vi "02_Stat_Read.vi"(1 "Command":T1(ring)) -> (0 "STAT":u32 format="%.0x")   [LabVIEW 2020]
panel:
  in  "Stat Array":bool[](array[boolean])=[FALSE, FALSE, FALSE, FALSE, FALSE, FALSE, FALSE, FALSE, FALSE, FALSE, FALSE, FALSE]
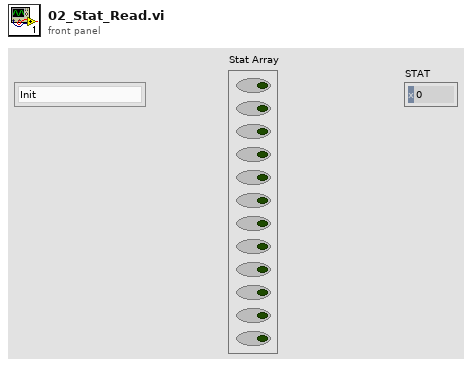
[diagram p1: front panel]
types:
  T1 = enum16{"Init", "Read", "Obs On", "Obs Off", "MStop On", "MStop Off"}
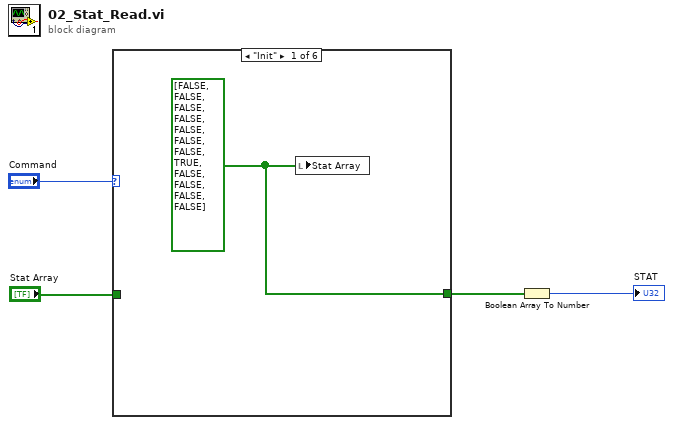
[diagram p0: block diagram]
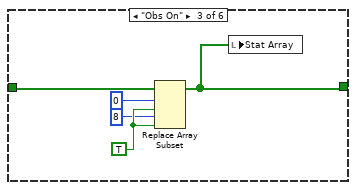
[diagram p3: hidden frame]
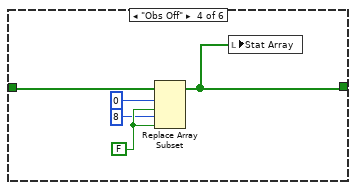
[diagram p4: hidden frame]
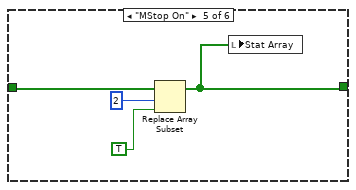
[diagram p5: hidden frame]
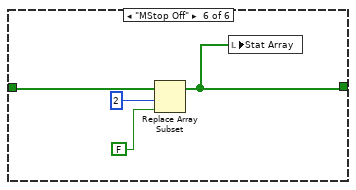
[diagram p6: hidden frame]
diagram:
  n1 = case shown="\"Init\"" "Command" {
    tunnel: "Stat Array" -> [_ w6 w8 w13 w18 w22]
    tunnel: [w5 w6 w7 w12 w17 w21] -> w2
    frame "Init" {
      w5 = bool[] [FALSE, FALSE, FALSE, FALSE, FALSE, FALSE, FALSE, TRUE, FALSE, FALSE, FALSE, FALSE] ("Stat Array")
      n2 = local write "Stat Array"(w5) -> ()
    }
    frame "Read" {
    }
    frame "Obs On" {
      w11 = TRUE ("new element/subarray")
      n3 = Replace Array Subset(array=w8, new element #1=w11, index #1=0 ("index"), new element #2=w11, index #2=8 ("index")) -> (w7:bool[])
      n4 = local write "Stat Array"(w7) -> ()
    }
    frame "Obs Off" {
      w16 = FALSE ("new element/subarray")
      n5 = Replace Array Subset(array=w13, new element #1=w16, index #1=0 ("index"), new element #2=w16, index #2=8 ("index")) -> (w12:bool[])
      n6 = local write "Stat Array"(w12) -> ()
    }
    frame "MStop On" {
      n7 = Replace Array Subset(array=w18, new element=TRUE ("new element/subarray"), index=2) -> (w17:bool[])
      n8 = local write "Stat Array"(w17) -> ()
    }
    frame "MStop Off" {
      n9 = Replace Array Subset(array=w22, new element=FALSE ("new element/subarray"), index=2) -> (w21:bool[])
      n10 = local write "Stat Array"(w21) -> ()
    }
  }
  n11 = Boolean Array To Number(Boolean array=w2) -> (number=→"STAT":u32)
